vi "RP Read RX FIFO Fast VISA.vi"(6 "Samples per read":i32=1024, 7 "bytes per sample":i32=12, 8 "Error In":errorcluster, 11 "VISA resource":refnum<visa-resource-name>) -> (0 "Error Out":errorcluster, 2 "FIFO out":i32[](array[numeric]), 3 "VISA resource out":refnum<visa-resource-name>)   [LabVIEW 2019]
uses:
  RP Command.ctl
  RP Write Command VISA.vi
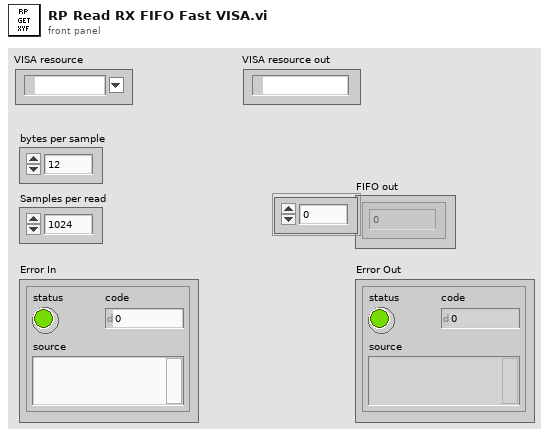
[diagram p1: front panel]
types:
  T1 = typedef "RP Command.ctl" = enum16{"Reset", "Read IDN", "Stop server", "Get status", "Get temperature", "Connect client", "Arm", "Software trigger", "Get whole buffer", "Get chunk", "System call", "Get config", "Set config", "Recieve data", "Recieve Calibartion", "Transmit data"}
  T2 = enum16{"big-endian, network order", "native, host order", "little-endian"}
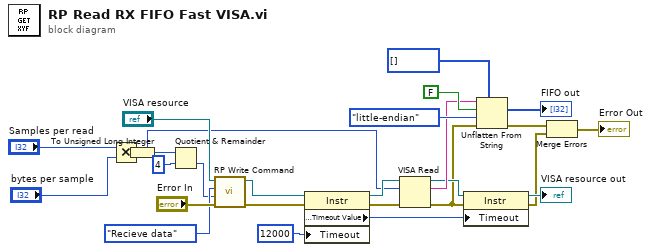
[diagram p0: block diagram]
diagram:
  n1 = Multiply(x="Samples per read", y="bytes per sample") -> (x*y=w13:i32)
  n2 = To Unsigned Long Integer(number=w13) -> (unsigned 32bit integer=w1:u32)
  n3 = Quotient & Remainder(x=w1, y=u32 4) -> (floor(x/y)=w16:u32)  [unwired: 1 out]
  n4 = call-poly "RP Write Command.vi"("Error In"="Error In", "Command payload"=w16, "Command number"=RP_Command."Recieve data", "VISA resource"="VISA resource") -> ("Error Out"=w6:errorcluster, "VISA resource out"=w12:refnum<visa-resource-name>)  [unwired: 5 in, 1 out]
  n5 = property class="Instr"(reference=w12, error in=w6, "Timeout"=u32 12000 ("timeout ms (25000)")) -> (reference out=w7:refnum<visa-resource-name>, error out=w5:errorcluster, "General Settings:Timeout Value"=w9:u32)
  n6 = VISA Read(VISA resource name=w7, byte count=w1, error in (no error)=w5) -> (VISA resource name out=w11:refnum<visa-resource-name>, read buffer=w14:string, error out=w4:errorcluster)  [unwired: 1 out]
  n7 = property class="Instr"(reference=w11, error in=w4, "Timeout"=w9) -> (reference out=→"VISA resource out":refnum<visa-resource-name>, error out=w2:errorcluster)
  n8 = Unflatten From String(type=i32[] [], binary string=w14, data includes array or string size? (T)=FALSE, byte order (0:big-endian, network order)=T2."little-endian", error in (no error)=w4) -> (value=→"FIFO out":i32[], error out=w22:errorcluster)  [unwired: 1 out]
  n9 = Merge Errors(w22, w2) -> (→"Error Out":errorcluster)
